vi "Open Excel Application.vi"(0 "Excel in":refnum<class "Excel.lvclass">, 1 "New instance? (false)":bool, 2 "Visible? (true)":bool=TRUE, 3 "error in (no error)":errorcluster, 4 "Alerts? (false)":bool) -> (7 "Excel out":refnum<class "Excel.lvclass">, 10 "error out":errorcluster)   [LabVIEW 2016, in "Excel.lvclass"]
uses:
  Excel.lvclass
  Excel.lvclass/Excel.ctl
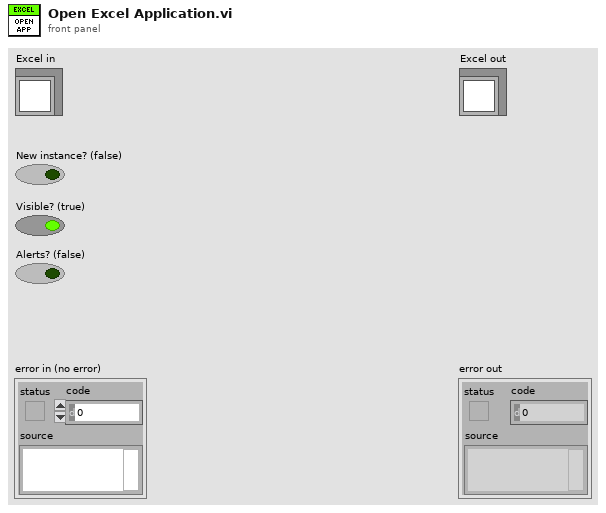
[diagram p1: front panel]
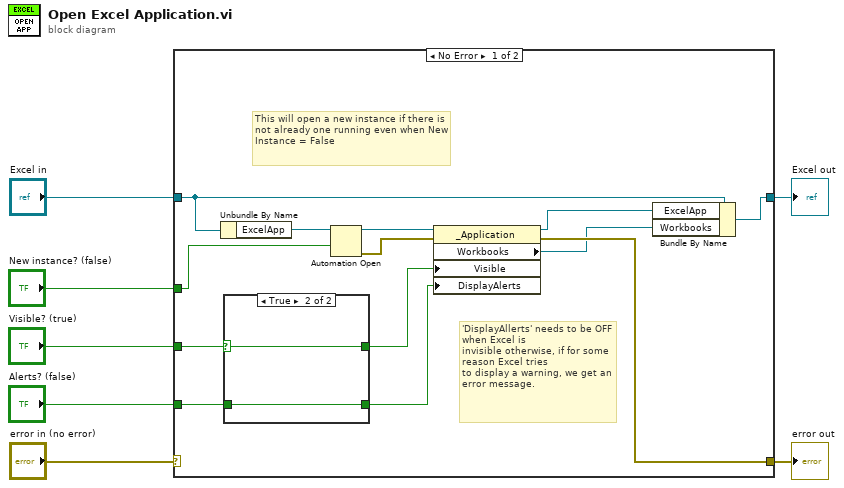
[diagram p0: block diagram]
diagram:
  n1 = case shown="No Error" "error in (no error)" {
    selector: "error in (no error)" -> [_ w25]
    tunnel: [w11 w25] -> w6
    tunnel: [w20 w24] -> w4
    tunnel: "Excel in" -> [w12 w24]
    tunnel: "New instance? (false)" -> [w17 _]
    tunnel: "Visible? (true)" -> [w16 _]
    tunnel: "Alerts? (false)" -> [w15 _]
    frame No Error {
      # "This will open a new instance if there is not already one running even when New Instance = False"
      # "'DisplayAllerts' needs to be OFF when Excel is\ninvisible otherwise, if for some reason Excel tries\nto display a warning, we get an error message."
      n2 = Unbundle By Name(w12) -> ("ExcelApp"=w19:refnum<k7>)
      n3 = case shown="True" w16 {
        selector: w16 -> [w21 w23]
        tunnel: [w21 w23] -> w14
        tunnel: w15 -> [_ w22]
        tunnel: [w21 w22] -> w13
        frame False {
        }
        frame True {
        }
      }
      n4 = Automation Open(Automation Refnum=w19, 9:w17) -> (Automation Refnum=w9:refnum<k7>, error out=w18:errorcluster)  [unwired: 2 in]
      n5 = property class="_Application"(reference=w9, error in=w18, "Visible"=w14, "DisplayAlerts"=w13) -> (reference out=w8:refnum<k7>, error out=w11:errorcluster, "Workbooks"=w10:refnum<k7>)
      n6 = Bundle By Name(cluster=w12, "ExcelApp"=w8, "Workbooks"=w10) -> (w20:refnum<class "Excel.lvclass">)
    }
    frame Error {
    }
  }
  "error out" <- w6
  "Excel out" <- w4
